vi "例4.10-1 累加（while循环）.vi"() -> ()   [LabVIEW 2017]
panel:
  out "和":i32
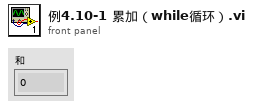
[diagram p1: front panel]
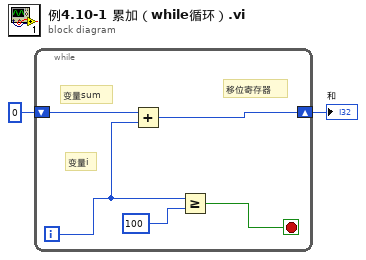
[diagram p0: block diagram]
diagram:
  n1 = while {
    shift-right: [w3] -> w1
    shift-left: 0 -> [w5]
    i -> [w4]
    stop <- w6 stop-if-true
    # "移位寄存器"
    # "变量i"
    # "变量sum"
    n2 = Add(x=w5, y=w4) -> (x+y=w3:i32)
    n3 = Greater Or Equal?(x=w4, y=100) -> (x >= y?=w6:bool)
  }
  "和" <- w1
